vi "__set_fieldCurrent_(Magnet_Current_Set2).vi"(6 "I mA":dbl=0.2362 step=2e-05, 7 "GPIB address of \nCurrent Source":string="25") -> ()   [LabVIEW 2013]
panel:
  in  "Case Constant\n(See Context Help)":bool=TRUE
  out "Present I (mA)":dbl=0.2362
  out "error out 2":errorcluster
  in  "error in (no error) 2":errorcluster
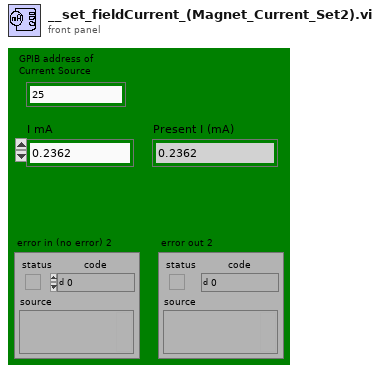
[diagram p1: front panel]
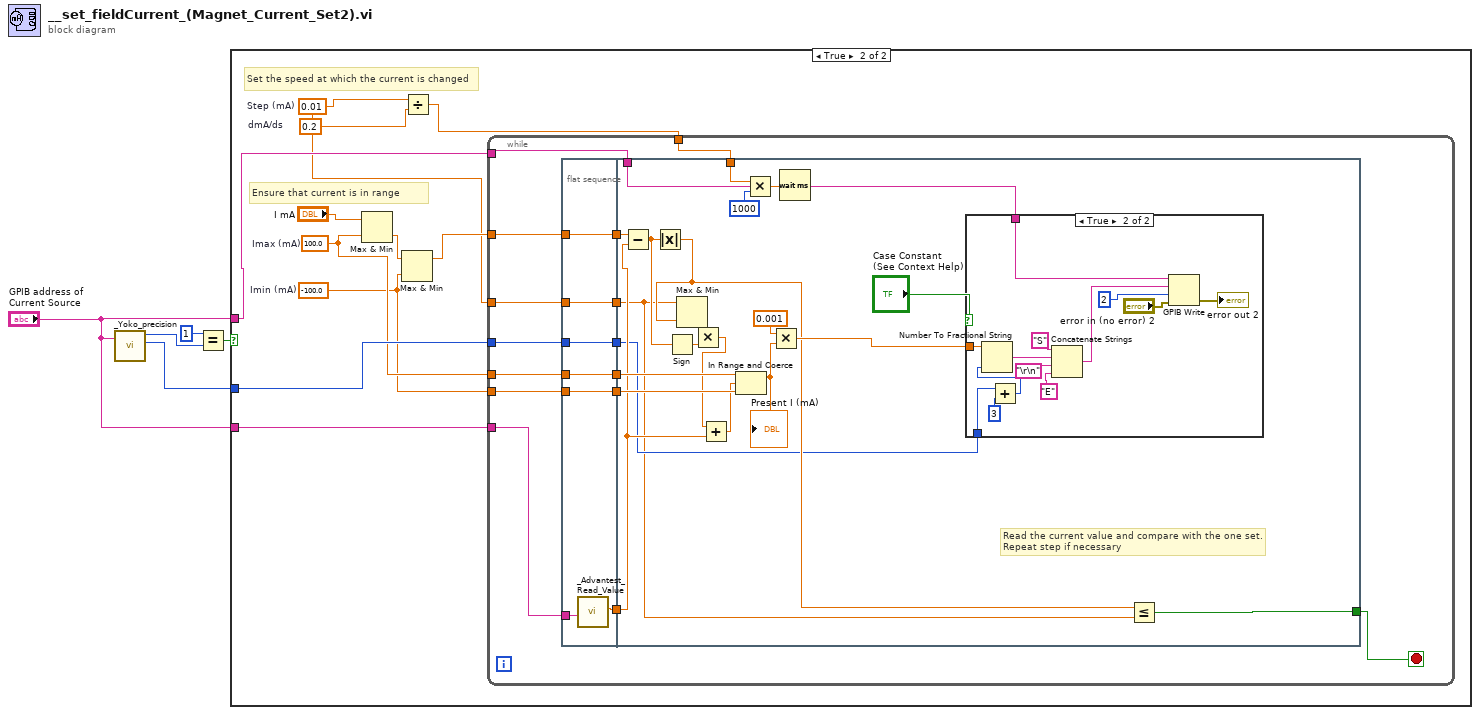
[diagram p0: block diagram]
diagram:
  n1 = call "_Yoko_precision.vi"("GPIB address (19)"="GPIB address of \nCurrent Source") -> ("Precision"=w3:i16, "Regime"=w1:i16)  [unwired: 3 in, 1 out]
  n2 = Equal?(x=1, y=w1) -> (x = y?=w5:bool)
  n3 = case shown="True" w5 {
    tunnel: "GPIB address of \nCurrent Source" -> [_ w16]
    tunnel: "GPIB address of \nCurrent Source" -> [_ w15]
    tunnel: w3 -> [_ w14]
    frame False {
    }
    frame True {
      w8 = 0.2  # dmA/ds
      w7 = 0.01  # Step (mA)
      w10 = 100.0  # Imax (mA)
      w9 = -100.0  # Imin (mA)
      # "Set the speed at which the current is changed"
      # "Ensure that current is in range"
      n4 = Max & Min(x="I mA", y=w10) -> (min(x,y)=w13:dbl)  [unwired: 1 out]
      n5 = Max & Min(x=w13, y=w9) -> (max(x,y)=w12:dbl)  [unwired: 1 out]
      n6 = Divide(x=w7, y=w8) -> (x/y=w6:dbl)
      n7 = while {
        tunnel: w6 -> [w31]
        tunnel: w7 -> [w30]
        tunnel: w12 -> [w27]
        tunnel: w10 -> [w29]
        tunnel: w9 -> [w28]
        tunnel: w16 -> [w25]
        tunnel: w15 -> [w20]
        tunnel: w14 -> [w18]
        stop <- w26 stop-if-true
        n8 = flat-sequence {
          tunnel: w27 -> [w35]
          tunnel: w28 -> [w36]
          tunnel: w29 -> [w37]
          tunnel: w30 -> [w38]
          tunnel: [w38] -> w24
          tunnel: [w37] -> w23
          tunnel: [w36] -> w22
          tunnel: [w35] -> w21
          tunnel: w20 -> [w34]
          tunnel: [w33] -> w19
          tunnel: w18 -> [w32]
          tunnel: [w32] -> w17
          tunnel: w31 -> [w57]
          tunnel: [w42] -> w26
          tunnel: w25 -> [w45]
          tunnel: w24 -> [w40]
          tunnel: w23 -> [w54]
          tunnel: w22 -> [w53]
          tunnel: w21 -> [w47]
          tunnel: w19 -> [w44]
          tunnel: w17 -> [w41]
          frame #0 {
            n9 = call "_Advantest_Read_Value.vi"("GPIB address (19)"=w34) -> ("Numeric"=w33:dbl)  [unwired: 1 in, 4 out]
          }
          frame #1 {
            # "Read the current value and compare with the one set.\nRepeat step if necessary"
            n10 = Subtract(x=w47, y=w44) -> (x-y=w46:dbl)
            n11 = Absolute Value(x=w46) -> (abs(x)=w43:dbl)
            n12 = Sign(1:w46) -> (0:w49:dbl)
            n13 = Max & Min(x=w40, y=w43) -> (min(x,y)=w50:dbl)  [unwired: 1 out]
            n14 = Multiply(x=w50, y=w49) -> (x*y=w48:dbl)
            n15 = Add(x=w48, y=w44) -> (x+y=w51:dbl)
            n16 = In Range and Coerce(upper limit=w54, x=w51, lower limit=w53) -> (coerced(x)=w39:dbl)  [unwired: 1 out]
            "Present I (mA)" <- w39
            n17 = Multiply(x=w57, y=1000) -> (x*y=w58:dbl)
            n18 = Multiply(x=0.001, y=w39) -> (x*y=w52:dbl)
            n19 = Wait (ms)(milliseconds to wait=w58) -> ()  [unwired: 1 out]
            n20 = case shown="True" "Case Constant\n(See Context Help)" {
              tunnel: w52 -> [_ w64]
              tunnel: w45 -> [_ w63]
              tunnel: w41 -> [_ w62]
              frame False {
              }
              frame True {
                n21 = Add(x=w62, y=3) -> (x+y=w60:i32)
                n22 = Number To Fractional String(number=w64, precision (6)=w60) -> (F-format string=w68:string)  [unwired: 2 in]
                n23 = Concatenate Strings("S", w68, "\r\n", "E") -> (w65:string)
                n24 = GPIB Write(0:w63, 1:w65, 2:2, 3:"error in (no error) 2") -> (6:→"error out 2":errorcluster)  [unwired: 1 in, 1 out]
              }
            }
            n25 = Less Or Equal?(x=w43, y=w40) -> (x <= y?=w42:bool)
          }
        }
      }
    }
  }
